vi "Request Data JSON.vi"(8 "error in (no error)":errorcluster, 11 "GetInputKindList in":refnum<class "GetInputKindList.lvclass">) -> (0 "error out":errorcluster, 2 "Request Data JSON":string, 3 "GetInputKindList out":refnum<class "GetInputKindList.lvclass">)   [LabVIEW 2022 SP3, in "obs-websocket-lv.lvlib" / "GetInputKindList.lvclass"]
uses:
  GetInputKindList.lvclass
  GetInputKindList.lvclass/GetInputKindList.ctl
  <vilib>/IlluminatedG/lv-web-crypto/lv-json/JSON/JSON.lvlib
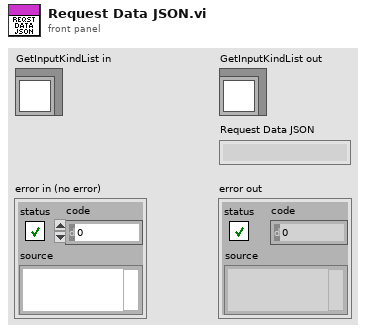
[diagram p1: front panel]
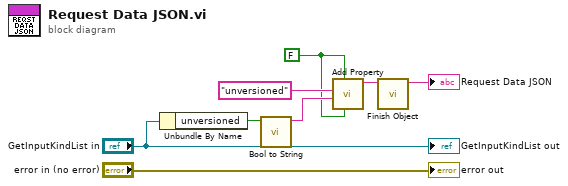
[diagram p0: block diagram]
diagram:
  w1 = FALSE ("Include Empty?")
  n1 = Unbundle By Name("GetInputKindList in") -> ("unversioned"=w5:bool)
  n2 = call <vilib>:"Bool to String.vi"("Boolean"=w5) -> ("Value"=w4:string)  [unwired: 10 in]
  n3 = call <vilib>:"Add Property.vi"("String?"=w1, "Include Empty?"=w1, "Value"=w4, "Property Name"="unversioned") -> ("String out"=w3:string)  [unwired: 7 in]
  n4 = call <vilib>:"Finish Object.vi"("String In"=w3) -> ("String out"=→"Request Data JSON":string)  [unwired: 10 in]
  "error out" <- "error in (no error)"
  "GetInputKindList out" <- "GetInputKindList in"
